vi "Create Subdirectories.vi"(8 "error in":errorcluster, 11 "Archivist in":refnum<class "Archivist.lvclass">) -> (0 "error out":errorcluster, 3 "Archivist out":refnum<class "Archivist.lvclass">)   [LabVIEW 2019, in "Archivist.lvclass"]
uses:
  Archivist.lvclass
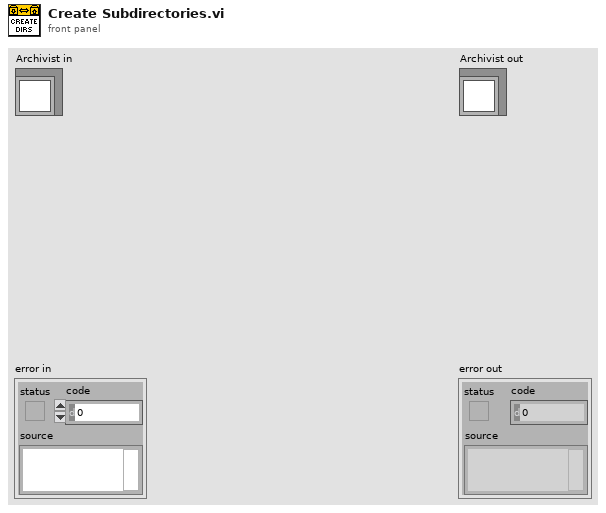
[diagram p1: front panel]
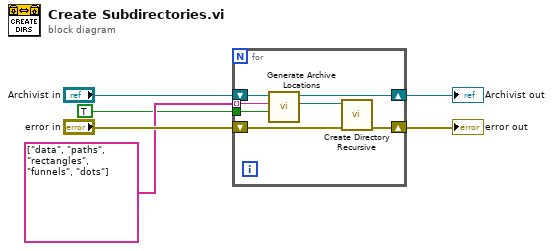
[diagram p0: block diagram]
diagram:
  n1 = for {
    shift-right: [w12] -> w5
    shift-left: "Archivist in" -> [w13]
    shift-right: [w10] -> w3
    shift-left: "error in" -> [w7]
    tunnel: string[] ["data", "paths", "rectangles", "funnels", "dots"] -> [w9] mode=indexing
    tunnel: TRUE ("Archive?") -> [w8]
    n2 = call "Generate Archive Locations.vi"("Archive?"=w8, "Key"=w9, "Archivist In"=w13) -> ("Path Out"=w11:path, "Archivist Out"=w12:refnum<class "Archivist.lvclass">)  [unwired: 7 in]
    n3 = call <vilib>:"Create Directory Recursive.vi"("error in (no error)"=w7, "directory"=w11) -> ("error out"=w10:errorcluster)  [unwired: 3 in, 2 out]
  }
  "error out" <- w3
  "Archivist out" <- w5
